vi "Find_Shift_Values.vi"(10 "Block":T1 {"orientaion" items=["up", "down", "left", "right"]; "type" items=["t", "rl", "ll", "rz", "lz", "square", "line"]}) -> (0 "y-value":dbl, 2 "x-value":dbl)   [LabVIEW 2015]
uses:
  block.ctl
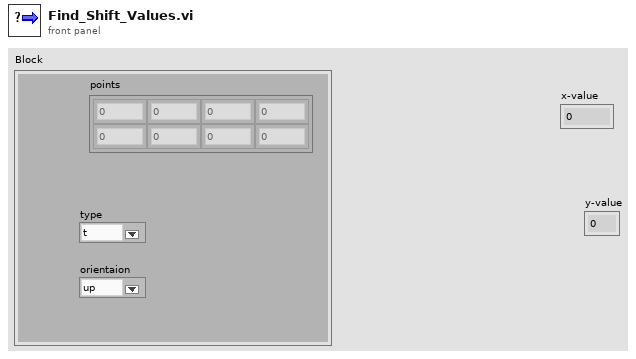
[diagram p1: front panel]
types:
  T1 = typedef "block.ctl" = cluster{"points":dbl[][], "type":u16, "orientaion":u16}
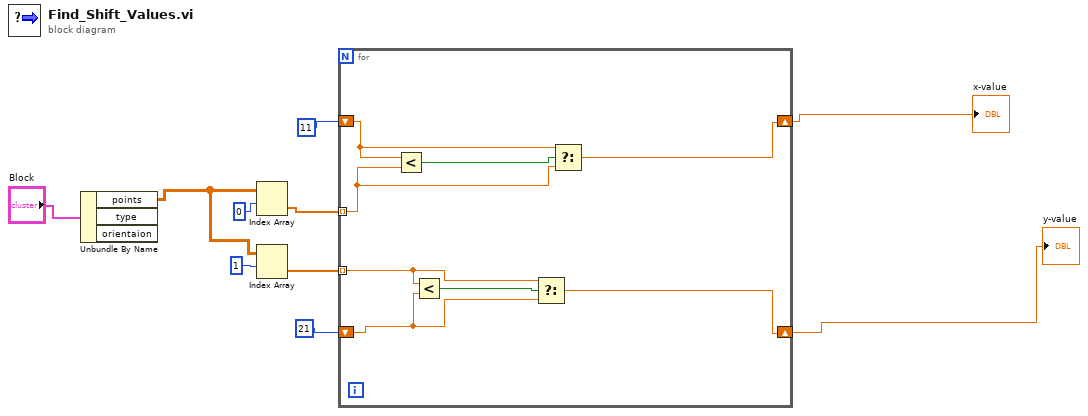
[diagram p0: block diagram]
diagram:
  n1 = Unbundle By Name("Block") -> ("points"=w8:dbl[][])  [unwired: 2 out]
  n2 = Index Array(array=w8, index (row)=0) -> (element=w6:dbl[])  [unwired: 1 in]
  n3 = Index Array(array=w8, index (row)=1) -> (element=w5:dbl[])  [unwired: 1 in]
  n4 = for {
    tunnel: w6 -> [w15] mode=indexing
    tunnel: w5 -> [w13] mode=indexing
    shift-right: [w11] -> w1
    shift-left: 21 -> [w12]
    shift-right: [w18] -> w2
    shift-left: 11 -> [w16]
    n5 = Less?(x=w16, y=w15) -> (x < y?=w17:bool)
    n6 = Less?(x=w13, y=w12) -> (x < y?=w14:bool)
    n7 = Select(t=w13, s=w14, f=w12) -> (s? t:f=w11:dbl)
    n8 = Select(t=w16, s=w17, f=w15) -> (s? t:f=w18:dbl)
  }
  "x-value" <- w2
  "y-value" <- w1
